vi "Create Coverage Report - Class Filename is VI Path.vi"() -> ()   [LabVIEW 2017, in "Cobertura.Tests.lvlib"]
uses:
  Cobertura.Tests.lvlib
  Fake Code Coverage/Fake Code Coverage.lvclass
  C:/Users/pasca/Projects/Home/lvunit/CodeCoverage/CodeCoverage.lvclass
  Fake Code Inspector/Fake Code Inspector.lvclass
  C:/Users/pasca/Projects/Home/lvunit/Cobertura/Code Inspector Base/Code Inspector Base.lvclass
  Cobertura/Coverage/Coverage.lvclass/Coverage.ctl
  Cobertura/Package/Package.lvclass/Package.ctl
  Cobertura/Class/Class.lvclass/Class.ctl
  Cobertura/Coverage/Read Packages.vi
  Cobertura/Package/Read Classes.vi
  Cobertura/Class/Read Filename.vi
  Fake Project Inspector/Fake Project Inspector.lvclass
  C:/Users/pasca/Projects/Home/lvunit/Cobertura/Project Inspector Base/Project Inspector Base.lvclass
  Cobertura/Package/Package.lvclass
  Cobertura/Class/Class.lvclass
  Cobertura/Cobertura.lvlib
  <vilib>/PNR/Transparent Assertions/Transparent Assertions/Transparent Assertions.lvlib
  Cobertura/Coverage/Coverage.lvclass
panel:
  out "error out":errorcluster
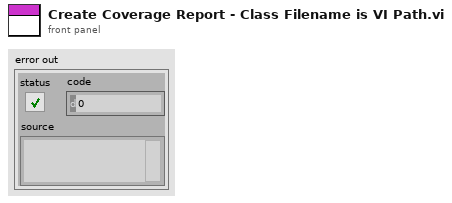
[diagram p1: front panel]
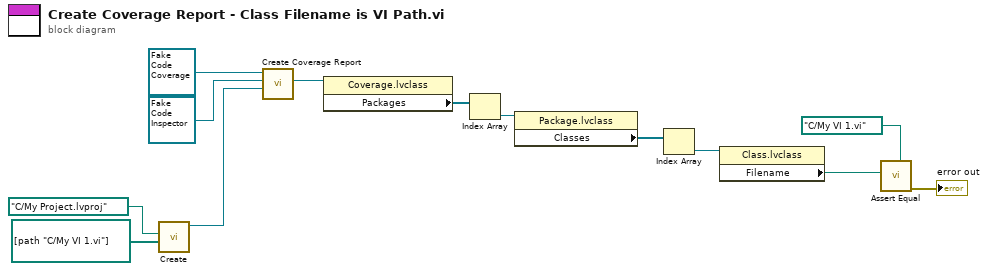
[diagram p0: block diagram]
diagram:
  n1 = call "Create.vi"("Item Paths"=path[] [path "C:/My VI 1.vi"], "Path"=path "C:/My Project.lvproj") -> ("Fake Project Inspector"=w8:refnum<class "Fake Project Inspector.lvclass">)  [unwired: 8 in, 1 out]
  n2 = call "Create Coverage Report.vi"("Project Inspector"=w8, "Code Inspector"=refnum<class "Fake Code Inspector.lvclass"> refnum ("Cobertura.Tests.lvlib:Fake Code Inspector.lvclass"), "CodeCoverage in"=refnum<class "Fake Code Coverage.lvclass"> refnum ("Cobertura.Tests.lvlib:Fake Code Coverage.lvclass")) -> ("Coverage"=w13:refnum<class "Coverage.lvclass">)  [unwired: 7 in, 1 out]
  n3 = property class="Coverage.lvclass"(reference=w13) -> ("Packages"=w11:refnum<class "Package.lvclass">[])  [unwired: 1 in, 2 out]
  n4 = Index Array(array=w11) -> (element=w6:refnum<class "Package.lvclass">)  [unwired: 1 in]
  n5 = property class="Package.lvclass"(reference=w6) -> ("Classes"=w5:refnum<class "Class.lvclass">[])  [unwired: 1 in, 2 out]
  n6 = Index Array(array=w5) -> (element=w3:refnum<class "Class.lvclass">)  [unwired: 1 in]
  n7 = property class="Class.lvclass"(reference=w3) -> ("Filename"=w2:path)  [unwired: 1 in, 2 out]
  n8 = call <vilib>:"Assert Equal.vi"("Expected"=path "C:/My VI 1.vi" ("Path"), "Actual"=w2) -> ("error out"=→"error out":errorcluster)  [unwired: 9 in]
